vi "Gas_Release_Control.vi"(4 "Establish Exp Conditions":bool, 6 "Strength (% by volume)":dbl format="%.3f", 7 "Carrier_2 Q (l/min)":dbl=20.0 format="%.2f", 8 "Carrier_1 Q (l/min)":dbl=20.0 format="%.2f", 9 "Source Status":T2) -> (0 "error out":errorcluster, 1 "Flowrates (kg/min)":dbl[](array[numeric]) format="%.2f", 2 "Source Est Time (s)":dbl, 3 "Flowrates Achieved?":bool)   [LabVIEW 2014]
uses:
  ADAM Controls/Client_Source_Status.ctl
  ADAM Controls/Client_Source.ctl
  ADAM Controls/Channel_names.ctl
  ADAM Controls/Module_type_ADAM.ctl
  ADAM Controls/Calib_type_ADAM.ctl
  ADAM Controls/Channel_State.ctl
  ADAM Controls/Ch_description_ADAM.ctl
  ADAM Controls/Function_ADAM.ctl
  ADAM Controls/Address.ctl
  ADAM Controls/Update_scan_value.ctl
  Anemometry/Anemometry Sub Vis/Controls/In_Range.ctl
  Anemometry/Anemometry Sub Vis/Globals/Preference_global.vi
panel:
  out "Q source":dbl
  out "Error String":string
  out "Currently on":T1=enum."Get Source Clients"
  out "Status of other Clients":string[](array[string])
  out "Source already correct?":bool
  out "No Other Clients are Using Source?":bool
  out "Source Clients":string[](array[string])
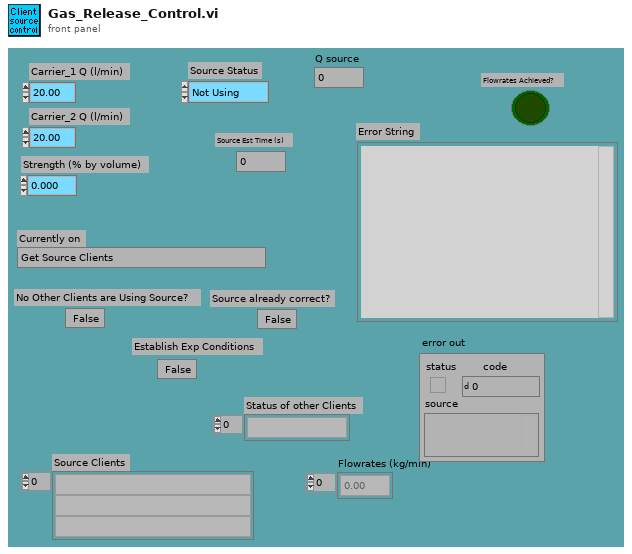
[diagram p1: front panel]
types:
  T1 = typedef "Client_Source.ctl" = enum16{"Start", "Get Source Clients", "Has this client liberty to control the source?", "Declare not using, other client already waiting", "Is the Source already correct?", "Declare waiting, other client is still using", "Control Hi-Tec", "Were the Hi-tecs able to achieve the flowrates?", "Declare source status", "Wait for source to Establish"}
  T2 = typedef "Client_Source_Status.ctl" = enum16{"Not Using", "Using", "Must Have"}
  T3 = typedef "Channel_names.ctl" = enum16{"Active Only", "Active + Off", "All Channels"}
  T4 = typedef "Ch_description_ADAM.ctl" = cluster{"Ch Name":string, "Type":T5, "Function":T6, "Ch State":T7, "Calibration type":T8, "A":dbl, "B":dbl, "C":dbl, "D":dbl, "Comments":string, "Address":T9, "String":string, "Duty":u16}
  T5 = typedef "Module_type_ADAM.ctl" = string
  T6 = typedef "Function_ADAM.ctl" = enum16{"Analogue Input", "Digital Input", "Event counter", "Event rate", "Analogue Output", "Digital Output", "Relay Output"}
  T7 = typedef "Channel_State.ctl" = enum16{"On", "Off", "Always On", "Always Off"}
  T8 = typedef "Calib_type_ADAM.ctl" = enum16{"Raw", "Bx + A", "Cx^2 + Bx + A", "Dx^3 + Cx^2 + Bx + A", "In Band", "Hi-Tec Q", "Hi-Tec M_dot", "Text"}
  T9 = typedef "Address.ctl" = cluster{"Main":i32, "Ch.":i32, "Sub":i32, "Port Name":string}
  T10 = typedef "Update_scan_value.ctl" = cluster{"Channel Name":string, "New Value":dbl}
  T11 = typedef "In_Range.ctl" = enum16{"%", "±", "% & ±"}
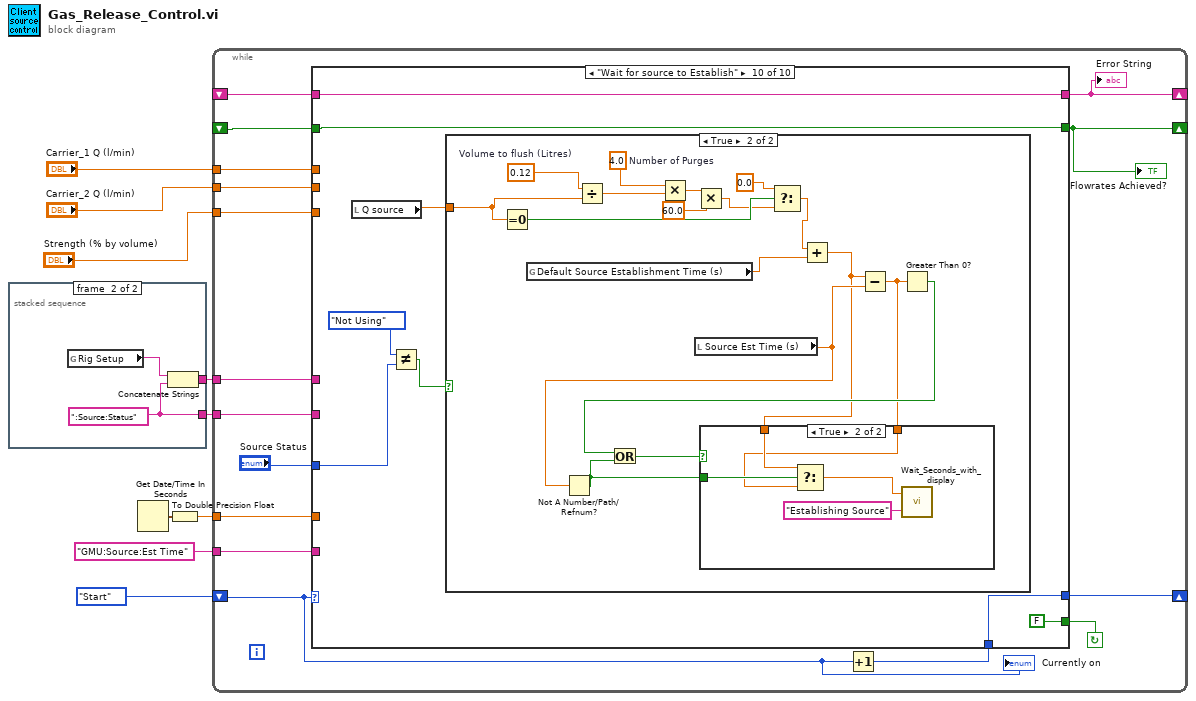
[diagram p0: block diagram]
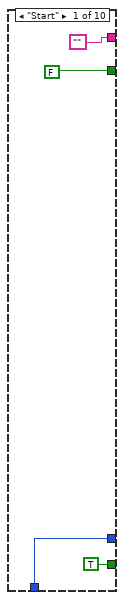
[diagram p2: hidden frame]
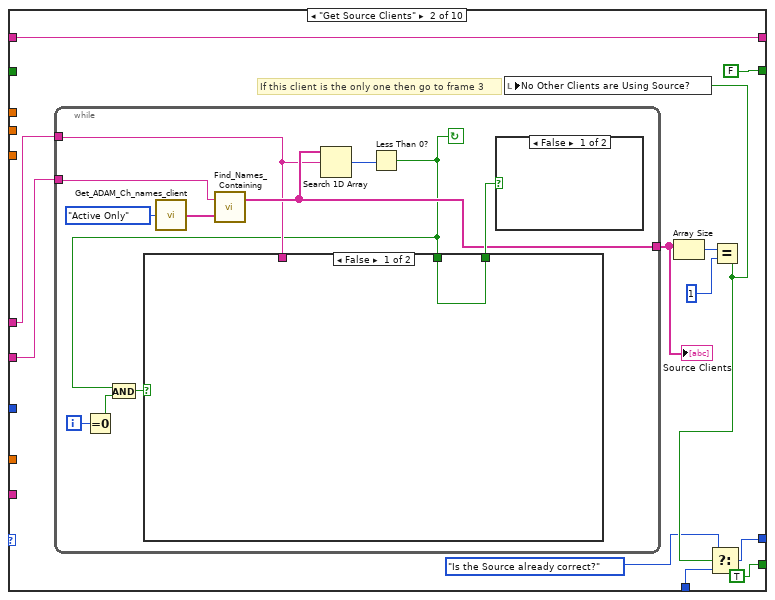
[diagram p3: hidden frame]
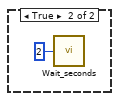
[diagram p4: hidden frame]
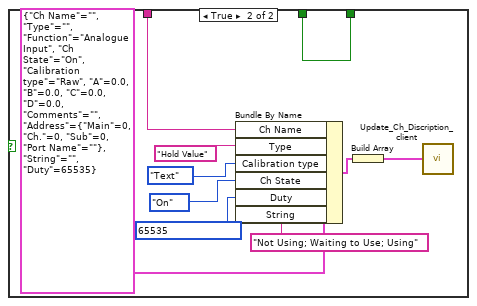
[diagram p5: hidden frame]
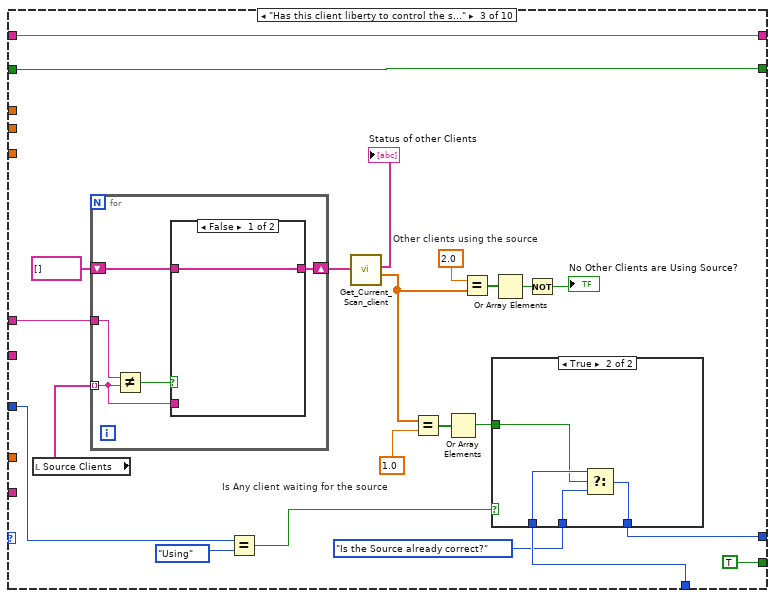
[diagram p6: hidden frame]
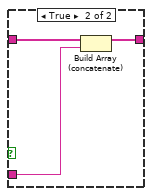
[diagram p8: hidden frame]
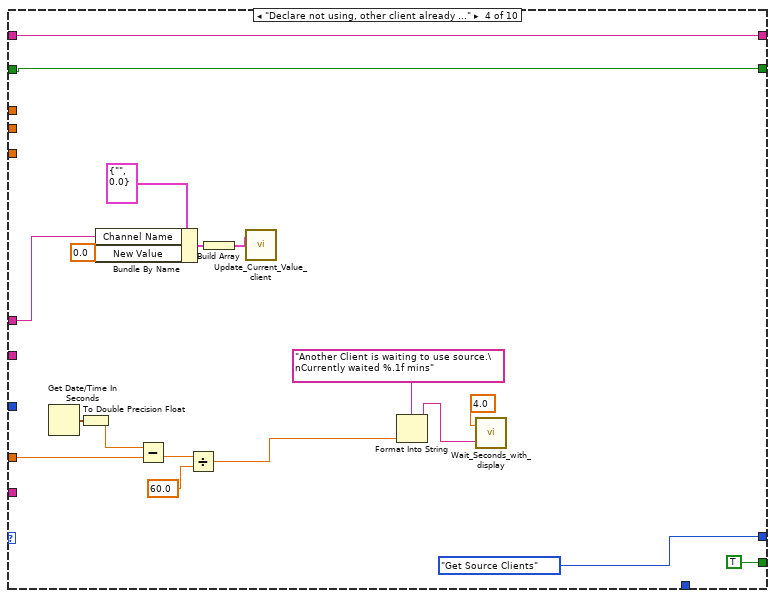
[diagram p9: hidden frame]
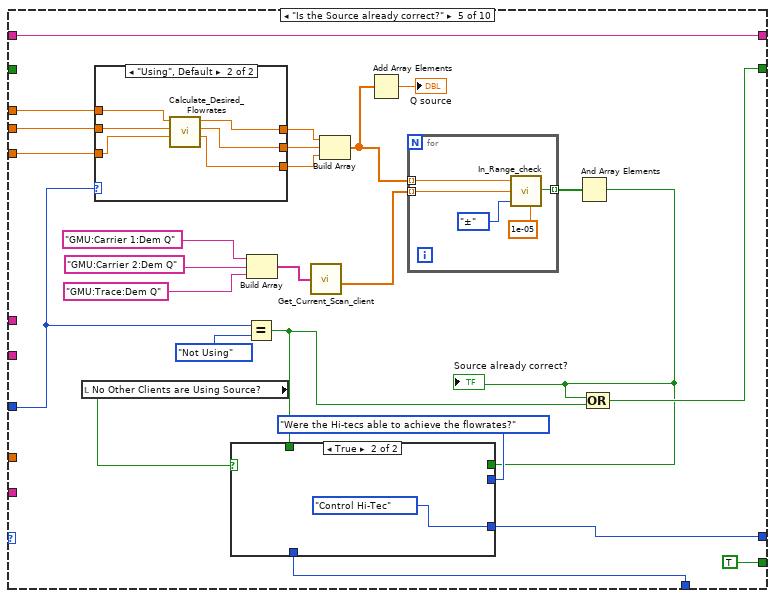
[diagram p10: hidden frame]
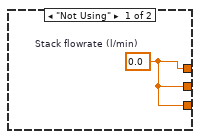
[diagram p11: hidden frame]
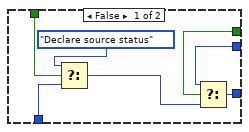
[diagram p12: hidden frame]
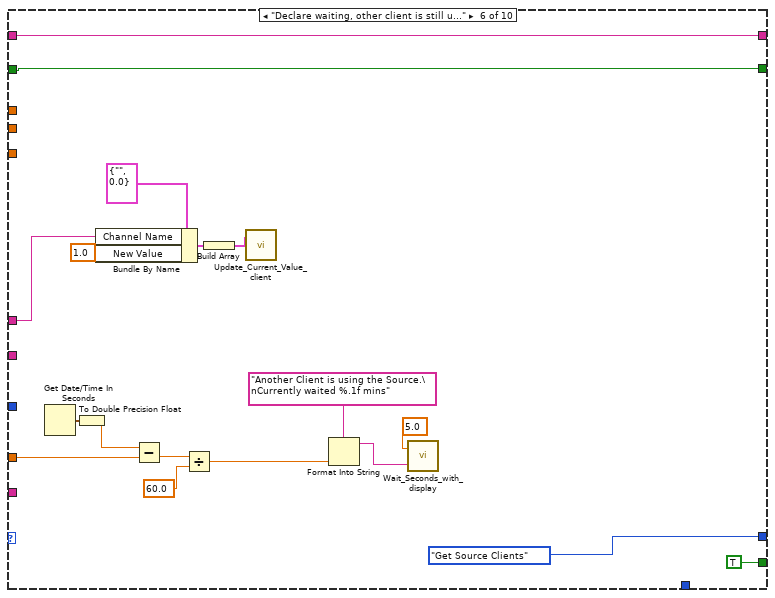
[diagram p13: hidden frame]
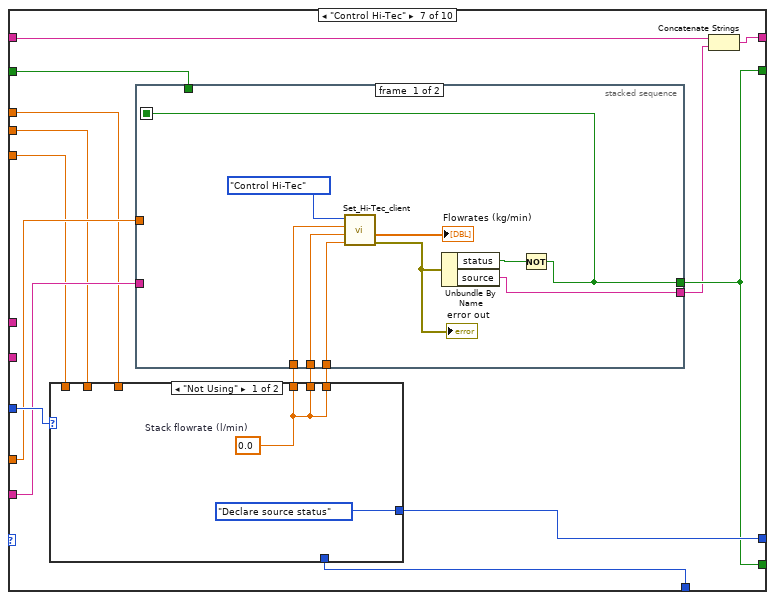
[diagram p14: hidden frame]
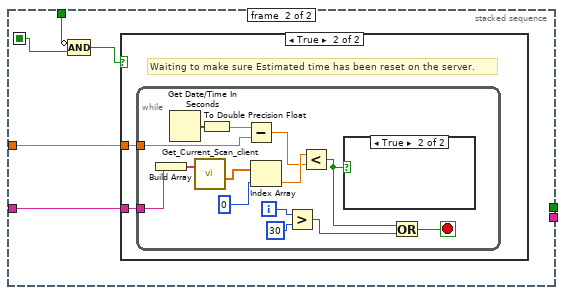
[diagram p15: hidden frame]
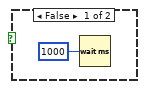
[diagram p17: hidden frame]
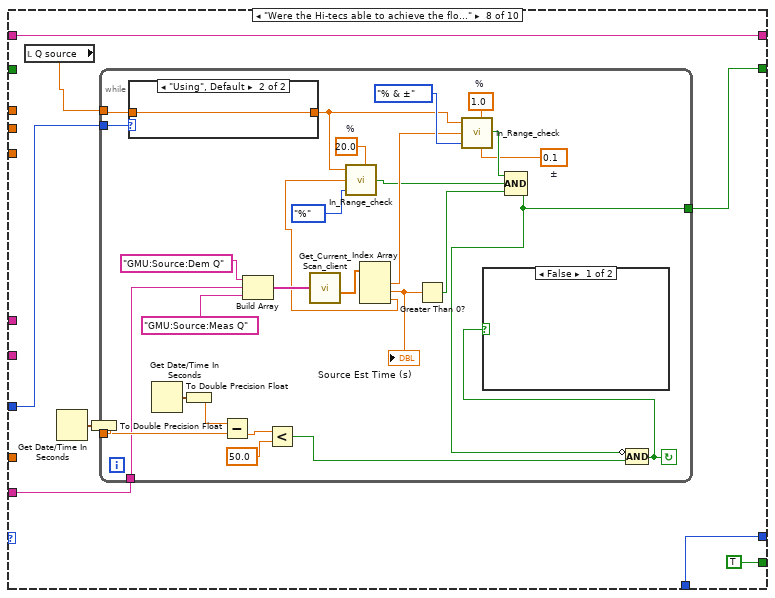
[diagram p19: hidden frame]
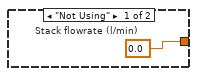
[diagram p20: hidden frame]
diagram:
  n1 = stacked-sequence {
    tunnel: [_ w12] -> w9
    tunnel: [_ w11] -> w8
    frame #0 {
      n2 = call "Run_EnFlo_Hub.vi"() -> ()  [unwired: 8 out]
    }
    frame #1 {
      w12 = ":Source:Status"
      n3 = global read "Preference_global.vi" "Rig Setup"() -> (w10:string)
      n4 = Concatenate Strings(w10, w12) -> (w11:string)
    }
  }
  n5 = Get Date/Time In Seconds() -> (seconds since 1Jan1904=w5:timestamp)
  n6 = To Double Precision Float(number=w5) -> (double precision float=w7:dbl)
  n7 = while {
    tunnel: w7 -> [w24]
    tunnel: w8 -> [w27]
    shift-left: Client_Source."Start" -> [w22]
    shift-right: [w23] -> _
    tunnel: w9 -> [w28]
    shift-right: [w19] -> _
    shift-left: _ -> [w20]
    tunnel: "GMU:Source:Est Time" -> [w18]
    shift-right: [w16] -> _
    shift-left: _ -> [w17]
    tunnel: "Carrier_1 Q (l/min)" -> [w15]
    tunnel: "Carrier_2 Q (l/min)" -> [w14]
    tunnel: "Strength (% by volume)" -> [w13]
    stop <- w26 continue-if-true
    n8 = Increment(x=w22) -> (x+1=w25:T1)
    n9 = case shown="\"Wait for source to Establish\"" w22 {
      tunnel: w28 -> [_ w44 _ _ _ _ _ _ _ _]
      tunnel: [w32 w40 w82 Client_Source."Get Source Clients" w134 Client_Source."Get Source Clients" w197 w244 w285 w306] -> w23
      tunnel: w27 -> [_ w43 w89 w116 _ w179 _ _ w287 _]
      tunnel: [TRUE ("Establish Exp Conditions") TRUE TRUE TRUE TRUE TRUE w193 TRUE w279 FALSE] -> w26
      tunnel: w25 -> [w32 w39 w84 _ w140 _ w196 w244 w285 w306]
      tunnel: w24 -> [_ _ _ w114 _ w174 w194 _ _ _]
      tunnel: "Source Status" -> [_ _ w73 _ w138 _ w200 w243 w286 w305]
      tunnel: [FALSE FALSE w69 w106 w136 w169 w193 w242 w280 w302] -> w19
      tunnel: w20 -> [_ _ w69 w106 _ w169 w192 _ w280 w302]
      tunnel: w18 -> [_ _ _ _ _ _ w195 w240 _ _]
      tunnel: w17 -> [_ w33 w68 w104 w133 w167 w190 w239 w278 w301]
      tunnel: ["" w33 w68 w104 w133 w167 w191 w239 w277 w301] -> w16
      tunnel: w15 -> [_ _ _ _ w126 _ w188 _ _ _]
      tunnel: w14 -> [_ _ _ _ w125 _ w187 _ _ _]
      tunnel: w13 -> [_ _ _ _ w124 _ w186 _ _ _]
      frame "Start" {
      }
      frame "Get Source Clients" {
        # "If this client is the only one then go to frame 3"
        n10 = while {
          tunnel: [w48] -> w37
          tunnel: w43 -> [w47]
          tunnel: w44 -> [w55]
          i -> [w52]
          stop <- w45 continue-if-true
          n11 = Equal To 0?(x=w52) -> (x = 0?=w51:bool)
          n12 = call "Get_ADAM_Ch_names_client.vi"("Channel names set"=Channel_names."Active Only") -> ("Ch names"=w53:string[])
          n13 = call "Find_Names_Containing.vi"("Ch names"=w53, "String to match"=w55) -> ("Matched Names"=w48:string[])  [unwired: 1 out]
          n14 = Search 1D Array(1D array=w48, element=w47) -> (index of element=w46:i32)  [unwired: 1 out]
          n15 = Less Than 0?(x=w46) -> (x < 0?=w45:bool)
          n16 = And(x=w45, y=w51) -> (x .and. y?=w50:bool)
          n17 = case shown="False" w50 {
            tunnel: w47 -> [_ w64]
            tunnel: [w57 w60] -> w49
            tunnel: w45 -> [w57 w60]
            frame False {
            }
            frame True {
              n18 = Bundle By Name(cluster=T4 {"Ch Name"="", "Type"="", "Function"=enum."Analogue Input", "Ch State"=enum."On", "Calibration type"=enum."Raw", "A"=0.0, "B"=0.0, "C"=0.0, "D"=0.0, "Comments"="", "Address"={"Main"=0, "Ch."=0, "Sub"=0, "Port Name"=""}, "String"="", "Duty"=65535} ("Ch Discription"), "Ch Name"=w64, "Type"=T5 "Hold Value", "Calibration type"=Calib_type_ADAM."Text", "Ch State"=Channel_State."On", "Duty"=u16 65535 ("Bundle Element"), "String"="Not Using; Waiting to Use; Using") -> (w62:T4)
              n19 = Build Array(w62) -> (w61:T4[])
              n20 = call "Update_Ch_Discription_client.vi"("Channels to update In"=w61) -> ()  [unwired: 1 out]
            }
          }
          n21 = case shown="False" w49 {
            frame False {
            }
            frame True {
              n22 = call "Wait_seconds.vi"("Seconds to wait"=u32 2) -> ()
            }
          }
        }
        "Source Clients" <- w37
        n23 = Array Size(array=w37) -> (size(s)=w42:i32)
        n24 = Equal?(x=w42, y=1) -> (x = y?=w36:bool)
        n25 = local write "No Other Clients are Using Source?"(w36) -> ()
        n26 = Select(t=Client_Source."Is the Source already correct?", s=w36, f=w39) -> (s? t:f=w40:T1)
      }
      frame "Has this client liberty to control the source?" {
        w81 = 2.0  # Other clients using the source
        w87 = 1.0  # Is Any client waiting for the source
        n27 = local read "Source Clients"() -> (w83:string[])
        n28 = for {
          tunnel: w83 -> [w95] mode=indexing
          tunnel: w89 -> [w99]
          shift-right: [w96] -> w79
          shift-left: string[] [] -> [w97]
          n29 = Not Equal?(x=w99, y=w95) -> (x != y?=w98:bool)
          n30 = case shown="False" w98 {
            tunnel: w97 -> [w100 w103]
            tunnel: [w100 w102] -> w96
            tunnel: w95 -> [_ w101]
            frame False {
            }
            frame True {
              n31 = Build Array (concatenate)(w103, w101) -> (w102:string[])
            }
          }
        }
        n32 = Equal?(x=w73, y=Client_Source_Status."Using" ("Source Status")) -> (x = y?=w72:bool)
        n33 = call "Get_Current_Scan_client.vi"("ADAM Ch Names"=w79) -> ("String values"=→"Status of other Clients":string[], "Numerical Values"=w76:dbl[])  [unwired: 2 out]
        n34 = Equal?(x=w76, y=w87) -> (x = y?=w86:bool[])
        n35 = Or Array Elements(Boolean array=w86) -> (logical OR=w77:bool)
        n36 = Equal?(x=w81, y=w76) -> (x = y?=w80:bool[])
        n37 = case shown="True" w72 {
          tunnel: w84 -> [_ w94]
          tunnel: [w90 w93] -> w82
          tunnel: w77 -> [_ w92]
          tunnel: Client_Source."Is the Source already correct?" -> [w90 w91]
          frame False {
          }
          frame True {
            n38 = Select(t=w94, s=w92, f=w91) -> (s? t:f=w93:T1)
          }
        }
        n39 = Or Array Elements(Boolean array=w80) -> (logical OR=w75:bool)
        n40 = Not(x=w75) -> (.not. x?=→"No Other Clients are Using Source?":bool)
      }
      frame "Declare not using, other client already waiting" {
        n41 = Get Date/Time In Seconds() -> (seconds since 1Jan1904=w105:timestamp)
        n42 = To Double Precision Float(number=w105) -> (double precision float=w115:dbl)
        n43 = Bundle By Name(cluster=T10 {"Channel Name"="", "New Value"=0.0} ("Update Scan Value Cluster"), "Channel Name"=w116, "New Value"=0.0 ("Bundle Element")) -> (w119:T10)
        n44 = Subtract(x=w115, y=w114) -> (x-y=w113:dbl)
        n45 = Divide(x=w113, y=60.0) -> (x/y=w107:dbl)
        n46 = Build Array(w119) -> (w118:T10[])
        n47 = call "Update_Current_Value_client.vi"("Update array in"=w118) -> ()  [unwired: 1 in]
        n48 = Format Into String(format string="Another Client is waiting to use source.\nCurrently waited %.1f mins" ("Format String"), w107) -> (resulting string=w110:string)  [unwired: 2 in, 1 out]
        n49 = call "Wait_Seconds_with_display.vi"("Message"=w110, "Seconds to wait"=4.0) -> ()  [unwired: 2 out]
      }
      frame "Is the Source already correct?" {
        n50 = local read "No Other Clients are Using Source?"() -> (w141:bool)
        n51 = case shown="\"Using\", Default" w138 {
          tunnel: [w152 w155] -> w131
          tunnel: [w152 w154] -> w130
          tunnel: [w152 w153] -> w129
          tunnel: w126 -> [_ w158]
          tunnel: w125 -> [_ w157]
          tunnel: w124 -> [_ w156]
          frame "Not Using" {
            w152 = 0.0  # Stack flowrate (l/min)
          }
          frame "Using", Default {
            n52 = call "Calculate_Desired_Flowrates.vi"("Strength (% by volume)"=w156, "Carrier_2 Q (l/min)"=w157, "Carrier_1 Q (l/min)"=w158) -> ("Trace Q l/min"=w153:dbl, "Carrier 2 l/min"=w154:dbl, "Carrier 1 l/min"=w155:dbl)  [unwired: 3 in, 2 out]
          }
        }
        n53 = Equal?(x=w138, y=Client_Source_Status."Not Using" ("Source Status")) -> (x = y?=w137:bool)
        n54 = Build Array("GMU:Carrier 1:Dem Q", "GMU:Carrier 2:Dem Q", "GMU:Trace:Dem Q") -> (w143:string[])
        n55 = call "Get_Current_Scan_client.vi"("ADAM Ch Names"=w143) -> ("Numerical Values"=w132:dbl[])  [unwired: 3 out]
        n56 = Build Array(w131, w130, w129) -> (w123:dbl[])
        n57 = Add Array Elements(numeric array=w123) -> (sum=→"Q source":dbl)
        n58 = for {
          tunnel: w132 -> [w149] mode=indexing
          tunnel: w123 -> [w148] mode=indexing
          tunnel: [w147] -> w128 mode=indexing
          n59 = call "In_Range_check.vi"("±"=1e-05, "Mode"=In_Range."±", "Value"=w149, "Setpoint"=w148) -> ("In Range"=w147:bool)  [unwired: 1 in, 2 out]
        }
        n60 = And Array Elements(Boolean array=w128) -> (logical AND=w127:bool)
        "Source already correct?" <- w127
        n61 = case shown="True" w141 {
          tunnel: w140 -> [w165 _]
          tunnel: w137 -> [w164 _]
          tunnel: w127 -> [w162 _]
          tunnel: Client_Source."Were the Hi-tecs able to achieve the flowrates?" -> [w160 _]
          tunnel: [w159 Client_Source."Control Hi-Tec"] -> w134
          frame False {
            n62 = Select(t=Client_Source."Declare source status", s=w164, f=w165) -> (s? t:f=w161:T1)
            n63 = Select(t=w160, s=w162, f=w161) -> (s? t:f=w159:T1)
          }
          frame True {
          }
        }
        n64 = Compound Arithmetic op=OR(w127, w137) -> (w136:bool)
      }
      frame "Declare waiting, other client is still using" {
        n65 = Get Date/Time In Seconds() -> (seconds since 1Jan1904=w168:timestamp)
        n66 = To Double Precision Float(number=w168) -> (double precision float=w177:dbl)
        n67 = Bundle By Name(cluster=T10 {"Channel Name"="", "New Value"=0.0} ("Update Scan Value Cluster"), "Channel Name"=w179, "New Value"=1.0 ("Bundle Element")) -> (w182:T10)
        n68 = Subtract(x=w177, y=w174) -> (x-y=w176:dbl)
        n69 = Divide(x=w176, y=60.0) -> (x/y=w170:dbl)
        n70 = Build Array(w182) -> (w181:T10[])
        n71 = call "Update_Current_Value_client.vi"("Update array in"=w181) -> ()  [unwired: 1 in]
        n72 = Format Into String(format string="Another Client is using the Source.\nCurrently waited %.1f mins" ("Format String"), w170) -> (resulting string=w173:string)  [unwired: 2 in, 1 out]
        n73 = call "Wait_Seconds_with_display.vi"("Message"=w173, "Seconds to wait"=5.0) -> ()  [unwired: 2 out]
      }
      frame "Control Hi-Tec" {
        n74 = case shown="\"Not Using\"" w200 {
          tunnel: [w232 w237] -> w199
          tunnel: w188 -> [_ w237]
          tunnel: [w232 w236] -> w198
          tunnel: w187 -> [_ w236]
          tunnel: [Client_Source."Declare source status" w235] -> w197
          tunnel: w196 -> [_ w235]
          tunnel: w186 -> [_ w234]
          tunnel: [w232 w234] -> w185
          frame "Not Using" {
            w232 = 0.0  # Stack flowrate (l/min)
          }
          frame "Using", Default {
          }
        }
        n75 = stacked-sequence {
          seq-local: [w203 _] -> [_ w212]
          tunnel: w199 -> [w207 _]
          tunnel: w198 -> [w206 _]
          tunnel: w195 -> [_ w214]
          tunnel: w194 -> [_ w213]
          tunnel: [w203 _] -> w193
          tunnel: w192 -> [_ w211]
          tunnel: [w202 _] -> w189
          tunnel: w185 -> [w201 _]
          frame #0 {
            n76 = call "Set_Hi-Tec_client.vi"("Strength (% by volume)"=w201, "Carrier_2 Q (l/min)"=w206, "Carrier_1 Q (l/min)"=w207, "Mode"=enum16{"Control Hi-Tec", "Check Hi-Tec Demands"}."Control Hi-Tec") -> ("error out"=w205:errorcluster, "Flowrates (kg/min)"=→"Flowrates (kg/min)":dbl[])  [unwired: 1 in, 3 out]
            "error out" <- w205
            n77 = Unbundle By Name(w205) -> ("status"=w204:bool, "source"=w202:string)
            n78 = Not(x=w204) -> (.not. x?=w203:bool)
          }
          frame #1 {
            n79 = Compound Arithmetic op=AND(invert w211, w212) -> (w210:bool)
            n80 = case shown="True" w210 {
              tunnel: w214 -> [_ w216]
              tunnel: w213 -> [_ w215]
              frame False {
              }
              frame True {
                # "Waiting to make sure Estimated time has been reset on the server."
                n81 = while {
                  tunnel: w216 -> [w229]
                  tunnel: w215 -> [w224]
                  i -> [w221]
                  stop <- w217 stop-if-true
                  n82 = Build Array(w229) -> (w230:string[])
                  n83 = Get Date/Time In Seconds() -> (seconds since 1Jan1904=w226:timestamp)
                  n84 = call "Get_Current_Scan_client.vi"("ADAM Ch Names"=w230) -> ("Numerical Values"=w228:dbl[])  [unwired: 3 out]
                  n85 = To Double Precision Float(number=w226) -> (double precision float=w225:dbl)
                  n86 = Subtract(x=w225, y=w224) -> (x-y=w222:dbl)
                  n87 = Index Array(array=w228, index=0) -> (element=w223:dbl)
                  n88 = Greater?(x=w221, y=30) -> (0:w218:bool)
                  n89 = Less?(x=w223, y=w222) -> (x < y?=w219:bool)
                  n90 = case shown="True" w219 {
                    frame False {
                      n91 = Wait (ms)(milliseconds to wait=u32 1000) -> ()  [unwired: 1 out]
                    }
                    frame True {
                    }
                  }
                  n92 = Or(x=w219, y=w218) -> (x .or. y?=w217:bool)
                }
              }
            }
          }
        }
        n93 = Concatenate Strings(w190, w189) -> (w191:string)
      }
      frame "Were the Hi-tecs able to achieve the flowrates?" {
        n94 = local read "Q source"() -> (w238:dbl)
        n95 = Get Date/Time In Seconds() -> (seconds since 1Jan1904=w241:timestamp)
        n96 = To Double Precision Float(number=w241) -> (double precision float=w245:dbl)
        n97 = while {
          tunnel: w243 -> [w262]
          tunnel: w238 -> [w261]
          tunnel: w245 -> [w271]
          tunnel: [w259] -> w242
          tunnel: w240 -> [w257]
          stop <- w268 continue-if-true
          w247 = 20.0  # %
          w260 = 0.1  # ±
          w266 = 1.0  # %
          n98 = case shown="\"Using\", Default" w262 {
            tunnel: [w274 w275] -> w249
            tunnel: w261 -> [_ w275]
            frame "Not Using" {
              w274 = 0.0  # Stack flowrate (l/min)
            }
            frame "Using", Default {
            }
          }
          n99 = Get Date/Time In Seconds() -> (seconds since 1Jan1904=w258:timestamp)
          n100 = To Double Precision Float(number=w258) -> (double precision float=w272:dbl)
          n101 = Subtract(x=w272, y=w271) -> (x-y=w248:dbl)
          n102 = Build Array("GMU:Source:Dem Q", w257, "GMU:Source:Meas Q") -> (w273:string[])
          n103 = Less?(x=w248, y=50.0) -> (x < y?=w269:bool)
          n104 = call "Get_Current_Scan_client.vi"("ADAM Ch Names"=w273) -> ("Numerical Values"=w264:dbl[])  [unwired: 3 out]
          n105 = Index Array(array=w264) -> (element #1=w252:dbl, element #2=w255:dbl, element #3=w253:dbl)  [unwired: 3 in]
          "Source Est Time (s)" <- w255
          n106 = call "In_Range_check.vi"("%"=w247, "Mode"=In_Range."%", "Value"=w253, "Setpoint"=w249) -> ("In Range"=w250:bool)  [unwired: 1 in, 2 out]
          n107 = Greater Than 0?(x=w255) -> (x > 0?=w251:bool)
          n108 = call "In_Range_check.vi"("±"=w260, "%"=w266, "Mode"=In_Range."% & ±", "Value"=w252, "Setpoint"=w249) -> ("In Range"=w263:bool)  [unwired: 2 out]
          n109 = Compound Arithmetic op=AND(w263, w250, w251) -> (w259:bool)
          n110 = Compound Arithmetic op=AND(invert w259, w269) -> (w268:bool)
          n111 = case shown="False" w268 {
            frame False {
            }
            frame True {
              n112 = Wait (ms)(milliseconds to wait=u32 1000) -> ()  [unwired: 1 out]
            }
          }
        }
      }
      frame "Declare source status" {
        n113 = case shown="True" w280 {
          tunnel: w286 -> [_ w296]
          tunnel: [0.0 w295] -> w281
          tunnel: [FALSE "Establish Exp Conditions"] -> w279
          tunnel: w278 -> [w289 w294]
          tunnel: [w288 w294] -> w277
          frame False {
            n114 = Concatenate Strings(w289, "Requested Flowrate has not been acheived.\n" ("Error String")) -> (w288:string)
          }
          frame True {
            n115 = case shown="\"Using\"" w296 {
              tunnel: [0.0 2.0 2.0] -> w295
              frame "Not Using" {
              }
              frame "Using" {
              }
              frame "Must Have" {
              }
            }
          }
        }
        n116 = Bundle By Name(cluster=T10 {"Channel Name"="", "New Value"=0.0} ("Update Scan Value Cluster"), "Channel Name"=w287, "New Value"=w281) -> (w283:T10)
        n117 = Build Array(w283) -> (w282:T10[])
        n118 = call "Update_Current_Value_client.vi"("Update array in"=w282) -> ()  [unwired: 1 in]
      }
      frame "Wait for source to Establish" {
        n119 = local read "Q source"() -> (w300:dbl)
        n120 = Not Equal?(x=Client_Source_Status."Not Using" ("Source Status"), y=w305) -> (x != y?=w303:bool)
        n121 = case shown="True" w303 {
          tunnel: w300 -> [_ w315]
          frame False {
          }
          frame True {
            w312 = 4.0  # Number of Purges
            w314 = 0.12  # Volume to flush (Litres)
            n122 = Equal To 0?(x=w315) -> (x = 0?=w318:bool)
            n123 = global read "Preference_global.vi" "Default Source Establishment Time (s)"() -> (w308:dbl)
            n124 = Divide(x=w314, y=w315) -> (x/y=w313:dbl)
            n125 = Multiply(x=w312, y=w313) -> (x*y=w311:dbl)
            n126 = local read "Source Est Time (s)"() -> (w320:dbl)
            n127 = Not A Number/Path/Refnum?(number/path/refnum=w320) -> (NaN/Path/Refnum?=w322:bool)
            n128 = Multiply(x=w311, y=60.0) -> (x*y=w309:dbl)
            n129 = Select(t=0.0, s=w318, f=w309) -> (s? t:f=w316:dbl)
            n130 = Add(x=w316, y=w308) -> (x+y=w319:dbl)
            n131 = Subtract(x=w319, y=w320) -> (x-y=w321:dbl)
            n132 = Greater Than 0?(x=w321) -> (x > 0?=w324:bool)
            n133 = Or(x=w324, y=w322) -> (x .or. y?=w323:bool)
            n134 = case shown="True" w323 {
              tunnel: w322 -> [_ w328]
              tunnel: w319 -> [_ w327]
              tunnel: w321 -> [_ w326]
              frame False {
              }
              frame True {
                n135 = Select(t=w327, s=w328, f=w326) -> (s? t:f=w325:dbl)
                n136 = call "Wait_Seconds_with_display.vi"("Message"="Establishing Source", "Seconds to wait"=w325) -> ()  [unwired: 2 out]
              }
            }
          }
        }
      }
    }
    "Flowrates Achieved?" <- w19
    "Error String" <- w16
    "Currently on" <- w22
  }
